vi "MSEncoder Act Execution.vi"(8 "error in (no error)":errorcluster, 11 "MSEncoder in":refnum<class "MSEncoder.lvclass">) -> (0 "error out":errorcluster, 3 "MSEncoder out":refnum<class "MSEncoder.lvclass">)   [LabVIEW 2018, in "MSEncoder.lvclass"]
uses:
  MSEncoder.lvclass
  MSEncoder.lvclass/MSEncoder.ctl
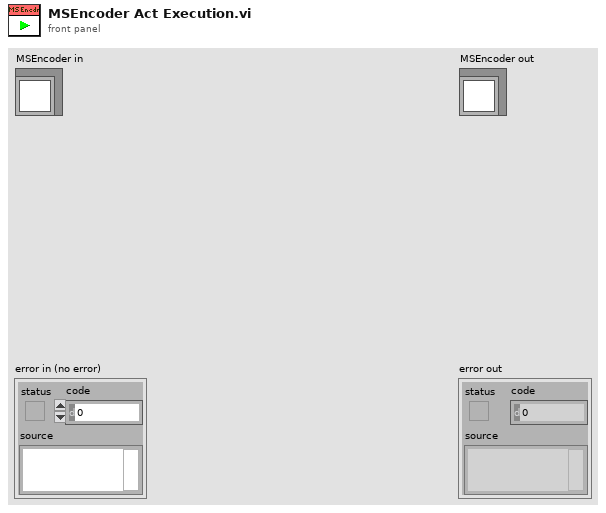
[diagram p1: front panel]
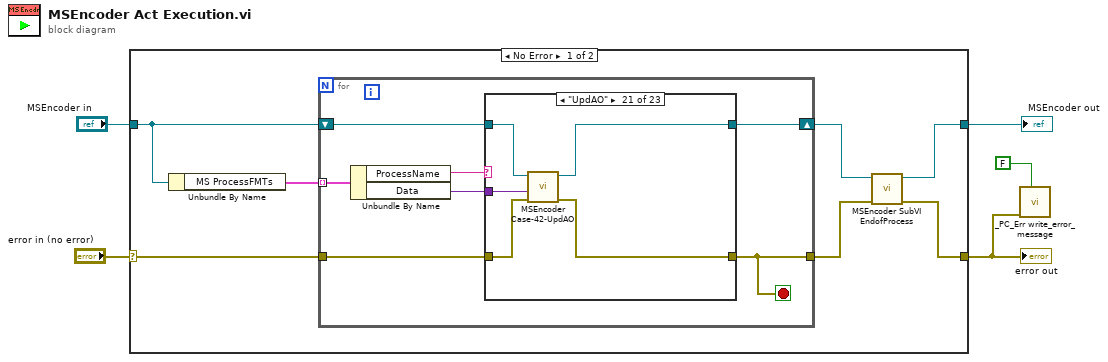
[diagram p0: block diagram]
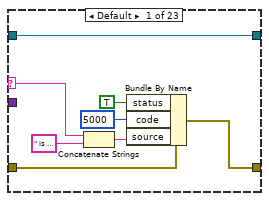
[diagram p2: hidden frame]
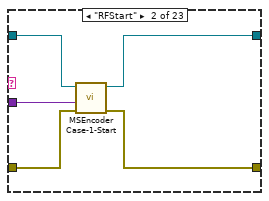
[diagram p3: hidden frame]
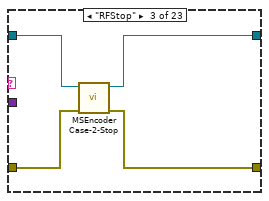
[diagram p4: hidden frame]
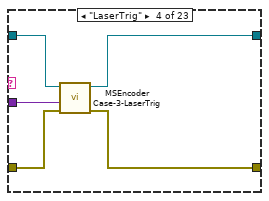
[diagram p5: hidden frame]
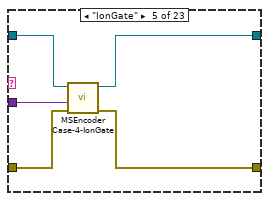
[diagram p6: hidden frame]
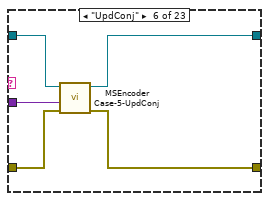
[diagram p7: hidden frame]
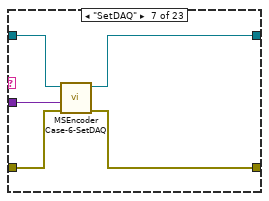
[diagram p8: hidden frame]
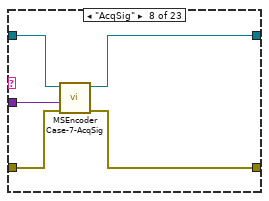
[diagram p9: hidden frame]
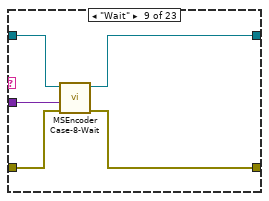
[diagram p10: hidden frame]
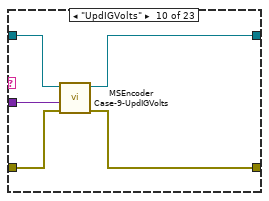
[diagram p11: hidden frame]
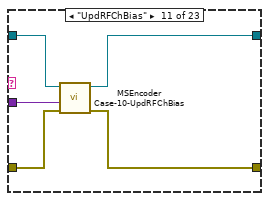
[diagram p12: hidden frame]
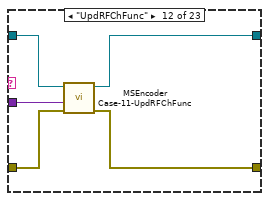
[diagram p13: hidden frame]
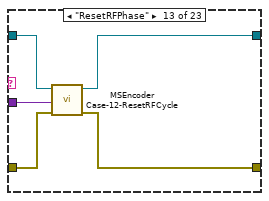
[diagram p14: hidden frame]
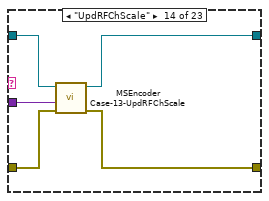
[diagram p15: hidden frame]
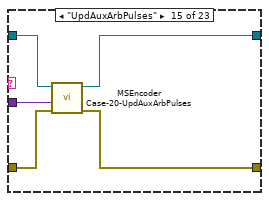
[diagram p16: hidden frame]
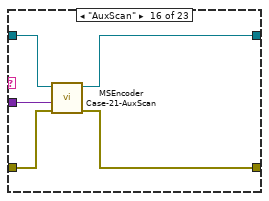
[diagram p17: hidden frame]
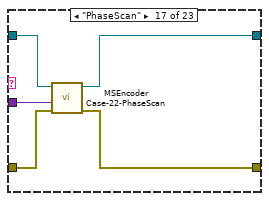
[diagram p18: hidden frame]
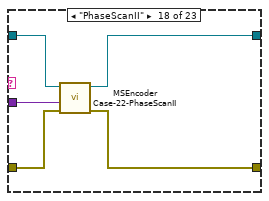
[diagram p19: hidden frame]
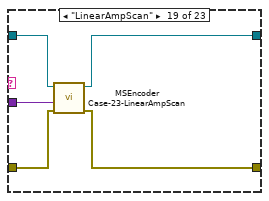
[diagram p20: hidden frame]
diagram:
  n1 = case shown="No Error" "error in (no error)" {
    selector: "error in (no error)" -> [w7 w138]
    tunnel: [w8 w138] -> w1
    tunnel: [w9 w137] -> w3
    tunnel: "MSEncoder in" -> [w12 w137]
    frame No Error {
      n2 = Unbundle By Name(w12) -> ("MS ProcessFMTs"=w11:cluster{"ProcessName":string, "Data":variant}[])
      n3 = for {
        shift-right: [w13] -> w10
        shift-left: w12 -> [w18]
        tunnel: w11 -> [w19] mode=indexing
        tunnel: w7 -> [w16]
        tunnel: [w15] -> w6
        stop <- w15 stop-if-true
        n4 = Unbundle By Name(w19) -> ("ProcessName"=w17:string, "Data"=w14:variant)
        n5 = case shown="\"UpdAO\"" w17 {
          selector: w17 -> [w22 _ _ _ _ _ _ _ _ _ _ _ _ _ _ _ _ _ _ _ _ _ _]
          tunnel: w18 -> [w27 w31 w35 w40 w45 w50 w55 w60 w63 w70 w75 w81 w82 w91 w95 w101 w105 w109 w115 w120 w126 w131 w135]
          tunnel: w16 -> [w26 w30 w34 w38 w43 w48 w53 w58 w64 w68 w73 w79 w84 w89 w93 w99 w103 w107 w112 w118 w123 w129 w133]
          tunnel: [w25 w29 w33 w39 w42 w47 w52 w57 w65 w67 w72 w77 w85 w88 w92 w98 w102 w110 w113 w117 w122 w127 w132] -> w15
          tunnel: w14 -> [_ w28 _ w37 w44 w49 w54 w59 w62 w69 w74 w80 w83 w90 w94 w100 w104 w108 w116 w119 w124 w130 w136]
          tunnel: [w27 w32 w36 w41 w46 w51 w56 w61 w66 w71 w76 w78 w86 w87 w96 w97 w106 w111 w114 w121 w125 w128 w134] -> w13
          frame Default {
            n6 = Concatenate Strings(w22, " is a undefined process to the MS encoder." ("source")) -> (w20:string)
            n7 = Bundle By Name(cluster=w26, "status"=TRUE, "code"=5000, "source"=w20) -> (w25:errorcluster)
          }
          frame "RFStart" {
            n8 = call "MSEncoder Case-1-Start.vi"("error in (no error)"=w30, "ParamValIn"=w28, "MSEncoder in"=w31) -> ("error out"=w29:errorcluster, "MSEncoder out"=w32:refnum<class "MSEncoder.lvclass">)  [unwired: 6 in, 1 out]
          }
          frame "RFStop" {
            n9 = call "MSEncoder Case-2-Stop.vi"("error in (no error)"=w34, "MSEncoder in"=w35) -> ("error out"=w33:errorcluster, "MSEncoder out"=w36:refnum<class "MSEncoder.lvclass">)  [unwired: 8 in]
          }
          frame "LaserTrig" {
            n10 = call "MSEncoder Case-3-LaserTrig.vi"("error in (no error)"=w38, "ParamValIn"=w37, "MSEncoder in"=w40) -> ("error out"=w39:errorcluster, "MSEncoder out"=w41:refnum<class "MSEncoder.lvclass">)  [unwired: 7 in]
          }
          frame "IonGate" {
            n11 = call "MSEncoder Case-4-IonGate.vi"("error in (no error)"=w43, "ParamValIn"=w44, "MSEncoder in"=w45) -> ("error out"=w42:errorcluster, "MSEncoder out"=w46:refnum<class "MSEncoder.lvclass">)  [unwired: 7 in]
          }
          frame "UpdConj" {
            n12 = call "MSEncoder Case-5-UpdConj.vi"("error in (no error)"=w48, "ParamValIn"=w49, "MSEncoder in"=w50) -> ("error out"=w47:errorcluster, "MSEncoder out"=w51:refnum<class "MSEncoder.lvclass">)  [unwired: 7 in]
          }
          frame "SetDAQ" {
            n13 = call "MSEncoder Case-6-SetDAQ.vi"("error in (no error)"=w53, "ParamValIn"=w54, "MSEncoder in"=w55) -> ("error out"=w52:errorcluster, "MSEncoder out"=w56:refnum<class "MSEncoder.lvclass">)  [unwired: 7 in]
          }
          frame "AcqSig" {
            n14 = call "MSEncoder Case-7-AcqSig.vi"("error in (no error)"=w58, "ParamValIn"=w59, "MSEncoder in"=w60) -> ("error out"=w57:errorcluster, "MSEncoder out"=w61:refnum<class "MSEncoder.lvclass">)  [unwired: 7 in]
          }
          frame "Wait" {
            n15 = call "MSEncoder Case-8-Wait.vi"("error in (no error)"=w64, "ParamValIn"=w62, "MSEncoder in"=w63) -> ("error out"=w65:errorcluster, "MSEncoder out"=w66:refnum<class "MSEncoder.lvclass">)  [unwired: 7 in]
          }
          frame "UpdIGVolts" {
            n16 = call "MSEncoder Case-9-UpdIGVolts.vi"("error in (no error)"=w68, "ParamValIn"=w69, "MSEncoder in"=w70) -> ("error out"=w67:errorcluster, "MSEncoder out"=w71:refnum<class "MSEncoder.lvclass">)  [unwired: 7 in]
          }
          frame "UpdRFChBias" {
            n17 = call "MSEncoder Case-10-UpdRFChBias.vi"("error in (no error)"=w73, "ParamValIn"=w74, "MSEncoder in"=w75) -> ("error out"=w72:errorcluster, "MSEncoder out"=w76:refnum<class "MSEncoder.lvclass">)  [unwired: 7 in]
          }
          frame "UpdRFChFunc" {
            n18 = call "MSEncoder Case-11-UpdRFChFunc.vi"("error in (no error)"=w79, "ParamValIn"=w80, "MSEncoder in"=w81) -> ("error out"=w77:errorcluster, "MSEncoder out"=w78:refnum<class "MSEncoder.lvclass">)  [unwired: 7 in]
          }
          frame "ResetRFPhase" {
            n19 = call "MSEncoder Case-12-ResetRFCycle.vi"("error in (no error)"=w84, "ParamValIn"=w83, "MSEncoder in"=w82) -> ("error out"=w85:errorcluster, "MSEncoder out"=w86:refnum<class "MSEncoder.lvclass">)  [unwired: 7 in]
          }
          frame "UpdRFChScale" {
            n20 = call "MSEncoder Case-13-UpdRFChScale.vi"("error in (no error)"=w89, "ParamValIn"=w90, "MSEncoder in"=w91) -> ("error out"=w88:errorcluster, "MSEncoder out"=w87:refnum<class "MSEncoder.lvclass">)  [unwired: 7 in]
          }
          frame "UpdAuxArbPulses" {
            n21 = call "MSEncoder Case-20-UpdAuxArbPulses.vi"("error in (no error)"=w93, "ParamValIn"=w94, "MSEncoder in"=w95) -> ("error out"=w92:errorcluster, "MSEncoder out"=w96:refnum<class "MSEncoder.lvclass">)  [unwired: 7 in]
          }
          frame "AuxScan" {
            n22 = call "MSEncoder Case-21-AuxScan.vi"("error in (no error)"=w99, "ParamValIn"=w100, "MSEncoder in"=w101) -> ("error out"=w98:errorcluster, "MSEncoder out"=w97:refnum<class "MSEncoder.lvclass">)  [unwired: 7 in]
          }
          frame "PhaseScan" {
            n23 = call "MSEncoder Case-22-PhaseScan.vi"("error in (no error)"=w103, "ParamValIn"=w104, "MSEncoder in"=w105) -> ("error out"=w102:errorcluster, "MSEncoder out"=w106:refnum<class "MSEncoder.lvclass">)  [unwired: 7 in]
          }
          frame "PhaseScanII" {
            n24 = call "MSEncoder Case-22-PhaseScanII.vi"("error in (no error)"=w107, "ParamValIn"=w108, "MSEncoder in"=w109) -> ("error out"=w110:errorcluster, "MSEncoder out"=w111:refnum<class "MSEncoder.lvclass">)  [unwired: 7 in]
          }
          frame "LinearAmpScan" {
            n25 = call "MSEncoder Case-23-LinearAmpScan.vi"("error in (no error)"=w112, "ParamValIn"=w116, "MSEncoder in"=w115) -> ("error out"=w113:errorcluster, "MSEncoder out"=w114:refnum<class "MSEncoder.lvclass">)  [unwired: 7 in]
          }
          frame "CLFreqScan" {
            n26 = call "MSEncoder Case-24-CLFreqScan.vi"("error in (no error)"=w118, "ParamValIn"=w119, "MSEncoder in"=w120) -> ("error out"=w117:errorcluster, "MSEncoder out"=w121:refnum<class "MSEncoder.lvclass">)  [unwired: 7 in]
          }
          frame "UpdAO" {
            n27 = call "MSEncoder Case-42-UpdAO.vi"("error in (no error)"=w123, "ParamValIn"=w124, "MSEncoder in"=w126) -> ("error out"=w122:errorcluster, "MSEncoder out"=w125:refnum<class "MSEncoder.lvclass">)  [unwired: 7 in]
          }
          frame "UpdDO" {
            n28 = call "MSEncoder Case-44-UpdDO.vi"("error in (no error)"=w129, "ParamValIn"=w130, "MSEncoder in"=w131) -> ("error out"=w127:errorcluster, "MSEncoder out"=w128:refnum<class "MSEncoder.lvclass">)  [unwired: 7 in]
          }
          frame "UpdFGen" {
            n29 = call "MSEncoder Case-45-FGen.vi"("error in (no error)"=w133, "ParamValIn"=w136, "MSEncoder in"=w135) -> ("error out"=w132:errorcluster, "MSEncoder out"=w134:refnum<class "MSEncoder.lvclass">)  [unwired: 7 in]
          }
        }
      }
      n30 = call "MSEncoder SubVI EndofProcess.vi"("error in (no error)"=w6, "MSEncoder in"=w10) -> ("error out"=w8:errorcluster, "MS Encoder"=w9:refnum<class "MSEncoder.lvclass">)  [unwired: 8 in]
    }
    frame Error {
    }
  }
  "error out" <- w1
  "MSEncoder out" <- w3
  n31 = call "_PC_Err write_error_message.vi"("show msg( T )"=FALSE, "error in"=w1) -> ()  [unwired: 9 in, 1 out]
